vi "Overwrite-all-hidden-params.vi"(8 "error in (no error)":errorcluster, 10 "Temp params adv":T1={"Axis origin relative position"=0.5, "Regression file relative path"=""}, 11 "Temp. params. ref. in":refnum<data-value>) -> (0 "error out":errorcluster, 3 "Temp. params. ref.":refnum<data-value>)   [LabVIEW 2013, in "CameraVision.lvlib" / "CV-Temperature.lvclass"]
uses:
  CV-Temperature.lvclass
  Temperature-parameters-advanced.ctl
  CV-Temperature.lvclass/CV-Temperature.ctl
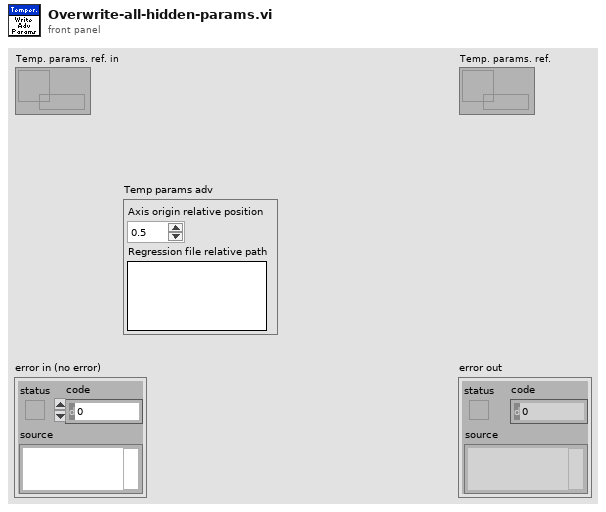
[diagram p1: front panel]
types:
  T1 = typedef "CameraVision.lvlib/CV-Temperature.lvclass/Temperature-parameters-advanced.ctl" = cluster{"Axis origin relative position":dbl, "Regression file relative path":string}
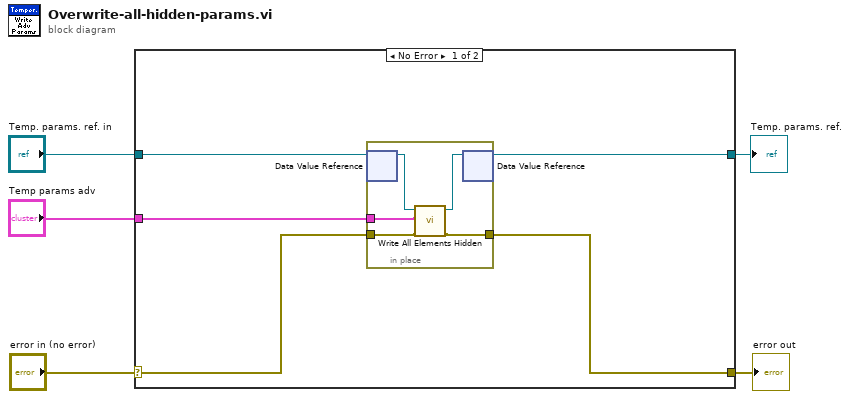
[diagram p0: block diagram]
diagram:
  n1 = case shown="No Error" "error in (no error)" {
    selector: "error in (no error)" -> [w8 w17]
    tunnel: [w9 w17] -> w4
    tunnel: "Temp. params. ref. in" -> [w7 w16]
    tunnel: "Temp params adv" -> [w10 _]
    tunnel: [w6 w16] -> w1
    frame No Error {
      n2 = in-place {
        in-place-border: w10 -> [w15]
        in-place-border: [w14] -> w9
        in-place-border: w8 -> [w13]
        n3 = in-place-dvr #1(w7) -> (w12:refnum<class "CV-Temperature.lvclass">)  [unwired: 1 out]
        n4 = call "Write All Elements Hidden.vi"("error in (no error)"=w13, "Temp. params. hidden"=w15, "Temp params in"=w12) -> ("error out"=w14:errorcluster, "Temp params out"=w11:refnum<class "CV-Temperature.lvclass">)  [unwired: 7 in]
        n5 = in-place-dvr #1(w11) -> (w6:refnum<data-value>)  [unwired: 1 out]
      }
    }
    frame Error {
    }
  }
  "error out" <- w4
  "Temp. params. ref." <- w1
